vi "Get Bouy.vi"(2 "error in":errorcluster, 3 "Image":T2) -> (0 "error out":errorcluster, 1 "Matches":T1[](array[typedef]) {"Correlation Score" format="%.2f"; "Target Template Curve Score" format="%.2f"; "Template Target Curve Score" format="%.2f"; "Bounding Box"."y" format="%.2f"; "Bounding Box"."x" format="%.2f"; "Position"."y" format="%.2f"; "Position"."x" format="%.2f"; "Score" format="%.2f"; "Scale" format="%.2f"; "Angle" format="%.2f"; "Occlusion %" format="%.2f"})   [LabVIEW 2011]
uses:
  <vilib>/vision/Image Controls.llb/IMAQ Image.ctl
  <vilib>/vision/Pattern Matching.llb/IMAQ GM Match Report.ctl
  <vilib>/vision/Pattern Matching.llb/IMAQ Curve Parameters.ctl
  <vilib>/vision/Pattern Matching.llb/IMAQ Match Range Setting.ctl
panel:
  in  "ROI Descriptor":T3={"Global Rectangle"=[127, 50, 551, 422], "Contours"=[{"ID"=enum."External", "Type"=12, "Coordinates"=[127, 50, 551, 422, 0]}]} {"Contours"."Type" items=["No Selection", "Point", "Line", "Rectangle", "Oval", "Polygon", "Freehand Region", "Annulus", "Unused2", "Unused3", "Broken Line", "Freehand Line", "Rotated Rectangle"]}
  out "Templete Image":T2(plugin-control)
  in  "Bouy\nTemplete":path=path "C:/Users/GARLAND/Documents/Projects/Robotics I/Robotics I 3390 2012/Final project/Labview/Pool navigation/bouy templete.png"
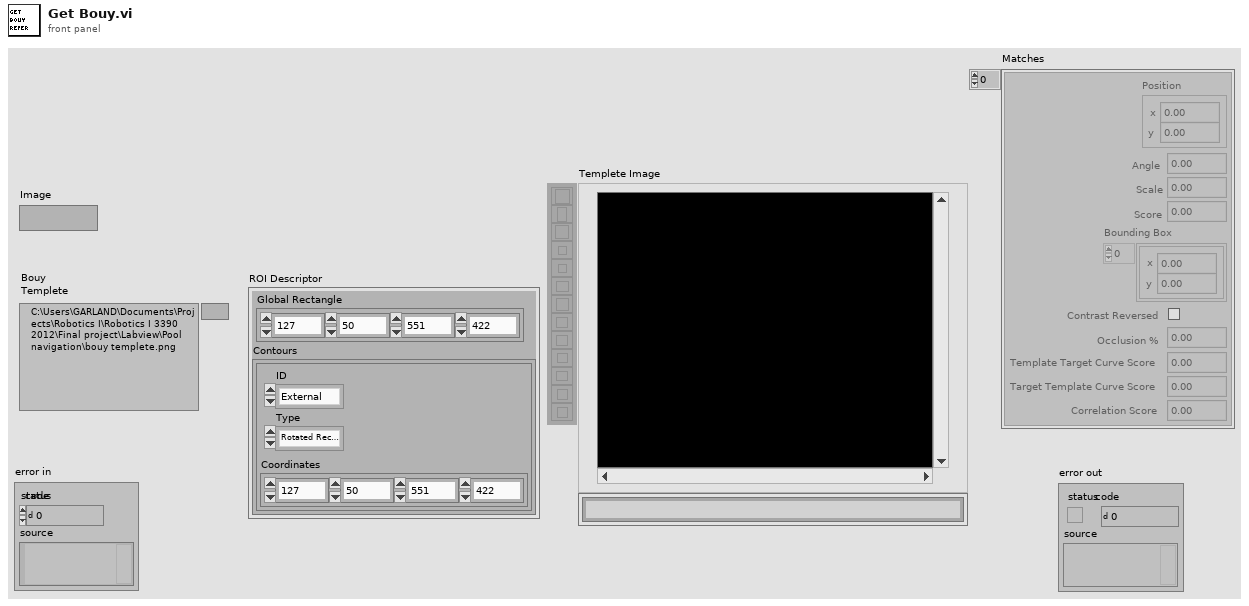
[diagram p1: front panel]
types:
  T1 = typedef "IMAQ GM Match Report.ctl" = cluster{"Position":cluster{"x":sgl, "y":sgl}, "Angle":sgl, "Scale":sgl, "Score":sgl, "Bounding Box":cluster{"x":sgl, "y":sgl}[], "Contrast Reversed":bool, "Occlusion %":sgl, "Template Target Curve Score":sgl, "Target Template Curve Score":sgl, "Correlation Score":sgl}
  T2 = typedef "IMAQ Image.ctl" = refnum<image>
  T3 = cluster{"Global Rectangle":i32[], "Contours":cluster{"ID":enum32{"External", "Internal"}, "Type":u32, "Coordinates":i32[]}[]}
  T4 = typedef "IMAQ Curve Parameters.ctl" = cluster{"Extraction Mode":u32, "Edge Threshold":i32, "Edge Filter Size":u32, "Min Length":i32, "Row Search Step Size":i32, "Col Search Step Size":i32, "Max Endpoint Gap":i32, "Closed":bool, "Subpixel":bool}
  T5 = typedef "IMAQ Match Range Setting.ctl" = cluster{"Match Constraints":u32, "Min":dbl, "Max":dbl}
  T6 = cluster{"Curve Parameters":T4, "Match Mode":cluster{"Rotation":bool, "Scale":bool, "Occlusion":bool, "Reserved":bool, "Reserved":bool, "Reserved":bool}, "Range Settings":T5[], "Number of Matches":i32, "Minimum Match Score":sgl, "SubPixel Accuracy":bool, "Adv. Geometric Match Options 2":cluster{"Setup Data Item":u16, "Item Value":dbl}[]}
  T7 = typedef "Image Type" = u32
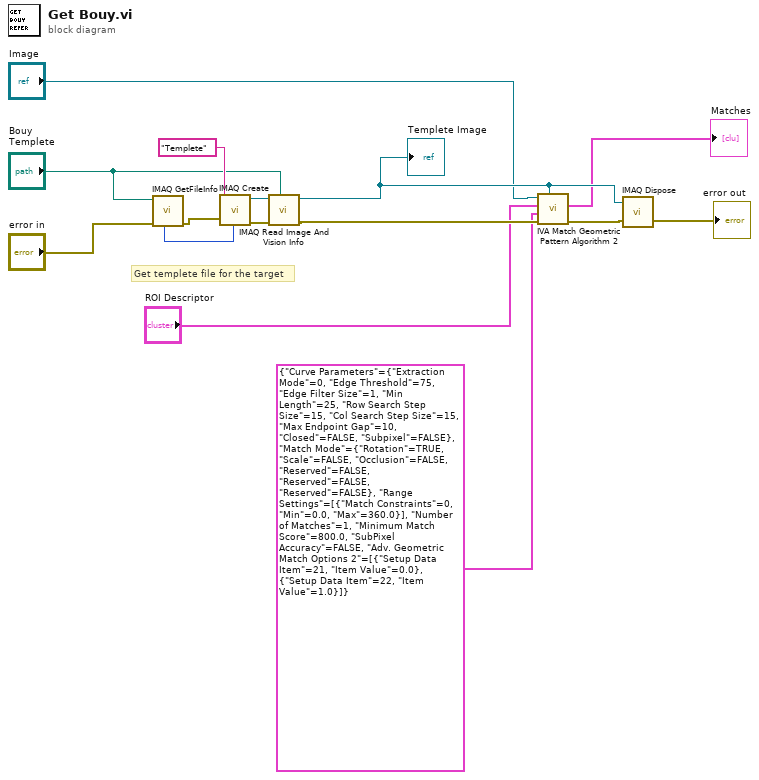
[diagram p0: block diagram]
diagram:
  # "Get templete file for the target"
  n1 = call "IMAQ GetFileInfo"("error in (no error)"="error in", "File Path"="Bouy\nTemplete") -> ("error out"=w13:errorcluster, "Image Type"=w12:T7)  [unwired: 3 in, 5 out]
  n2 = call "IMAQ Create"("Image Name"="Templete", "Image Type"=w12, "error in (no error)"=w13) -> ("New Image"=w15:T2, "error out"=w14:errorcluster)  [unwired: 1 in, 1 out]
  n3 = call "IMAQ Read Image And Vision Info"("File Path"="Bouy\nTemplete", "error in (no error)"=w14, "Image"=w15) -> ("error out"=w3:errorcluster, "Image Out"=w7:T2)  [unwired: 1 in, 6 out]
  "Templete Image" <- w7
  n4 = call <vilib>:"IVA Match Geometric Pattern Algorithm 2.vi"("Template"=w7, "error in (no error)"=w3, "Settings"=T6 {"Curve Parameters"={"Extraction Mode"=0, "Edge Threshold"=75, "Edge Filter Size"=1, "Min Length"=25, "Row Search Step Size"=15, "Col Search Step Size"=15, "Max Endpoint Gap"=10, "Closed"=FALSE, "Subpixel"=FALSE}, "Match Mode"={"Rotation"=TRUE, "Scale"=FALSE, "Occlusion"=FALSE, "Reserved"=FALSE, "Reserved"=FALSE, "Reserved"=FALSE}, "Range Settings"=[{"Match Constraints"=0, "Min"=0.0, "Max"=360.0}], "Number of Matches"=1, "Minimum Match Score"=800.0, "SubPixel Accuracy"=FALSE, "Adv. Geometric Match Options 2"=[{"Setup Data Item"=21, "Item Value"=0.0}, {"Setup Data Item"=22, "Item Value"=1.0}]}, "ROI Descriptor"="ROI Descriptor", "Image"="Image") -> ("error out"=w4:errorcluster, "Matches"=→"Matches":T1[])  [unwired: 1 in, 4 out]
  n5 = call "IMAQ Dispose"("Image"=w7, "error in (no error)"=w4) -> ("error out"=→"error out":errorcluster)  [unwired: 4 in]
